vi "Google - URL - Build (for stock ticker).vi"(0 "Symbol":string, 3 "error in":errorcluster) -> (6 "URL":string, 9 "error out":errorcluster)   [LabVIEW 2011]
doc: "Build the URL required to retrieve the stock data from Google Finance.\n\nInputs:\n Symbol: Stock ticker symbol.\n Error in: Describes error conditions that occur before this node runs. This input provides standard error in functionality.\n\nOutputs:\n URL: URL of the HTTP request.\n Error out: Contains error information. This output provides standard error out functionality."
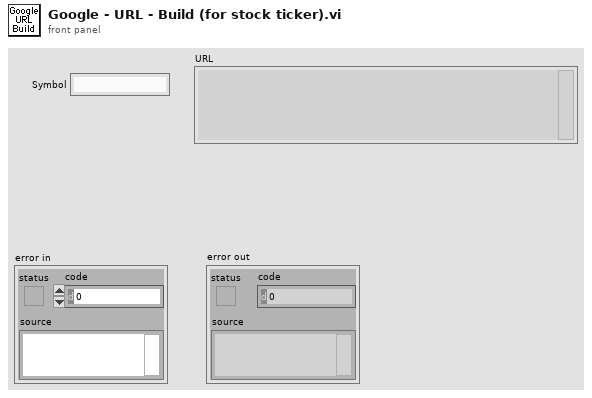
[diagram p1: front panel]
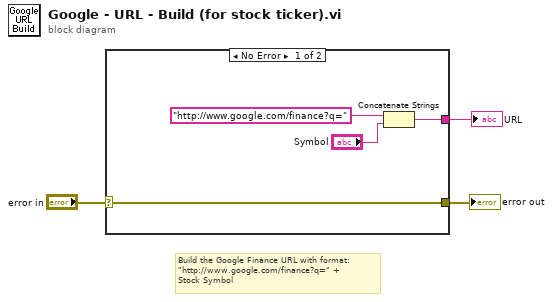
[diagram p0: block diagram]
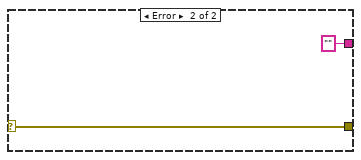
[diagram p2: hidden frame]
diagram:
  # "Build the Google Finance URL with format:\n\"http://www.google.com/finance?q=\" +\nStock Symbol"
  n1 = case shown="No Error" "error in" {
    selector: "error in" -> [w5 w9]
    tunnel: [w6 ""] -> w3
    tunnel: [w5 w9] -> w2
    frame No Error {
      n2 = Concatenate Strings("http://www.google.com/finance?q=" ("string"), "Symbol") -> (w6:string)
    }
    frame Error {
    }
  }
  "URL" <- w3
  "error out" <- w2
